vi "transition.vi"(8 "error in (no error)":errorcluster, 10 "Context In":refnum<class "ContextData.lvclass">, 11 "Wait Event in":refnum<class "Wait Event.lvclass">) -> (0 "error out":errorcluster, 2 "Context Out":refnum<class "ContextData.lvclass">, 3 "Next State":refnum<class "State.lvclass">)   [LabVIEW 2019, in "Wait Event.lvclass"]
uses:
  Wait Event.lvclass
  State/State.lvclass
  ContextData/ContextData.lvclass
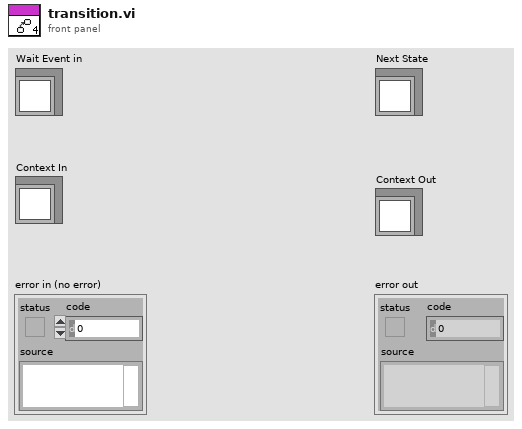
[diagram p1: front panel]
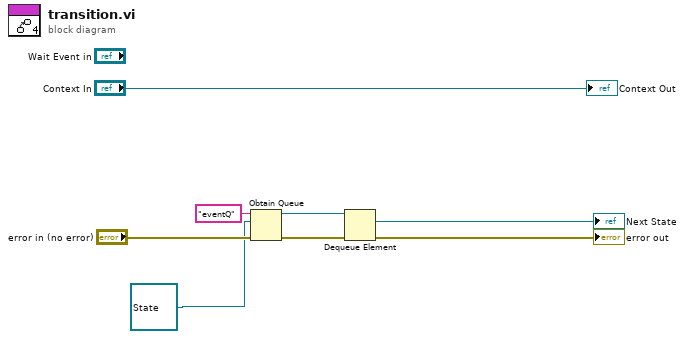
[diagram p0: block diagram]
diagram:
  n1 = Obtain Queue(name (unnamed)="eventQ", element data type=refnum<class "State.lvclass"> refnum ("Context DVR In"), error in (no error)="error in (no error)") -> (queue out=w5:refnum<queue>, error out=w7:errorcluster)  [unwired: 2 in, 1 out]
  n2 = Dequeue Element(queue=w5, error in (no error)=w7) -> (element=→"Next State":refnum<class "State.lvclass">, error out=→"error out":errorcluster)  [unwired: 1 in, 2 out]
  "Context Out" <- "Context In"
